vi "PCO_CheckDeviceAvailability.vi"(8 "error in (no error)":errorcluster {"code" format="%x"}, 10 "wNum":u16, 11 "ph":u64) -> (0 "error out":errorcluster {"code" format="%x"}, 2 "ErrorMessage":i32 format="%x", 3 "ph out":u64)   [LabVIEW 2019, in "SDK.lvlib" / "CameraAccess.lvlib"]
doc: "<b>Description:</b>\nThis function is used to check, if the connection to a previously opened camera is still valid. Functionality is only supported for interfaces with HotPlug capability like USB, GigE or FireWire.\nIf a device is connected or disconnected from a HotPlug capable bus system, the device manager does invoke a bus reset call on the bus and afterwards is starting a new enumeration. If enumeration is finished, a DEVICE_CHANGE message is broadcasted to all applications.\n\n<b>Supported camera type:</b>\nInterface dependent\n\n<b>Descriptor dependency:</b>\nNone"
uses:
  CameraAccess.lvlib
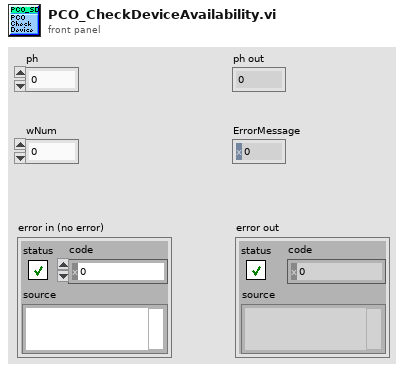
[diagram p1: front panel]
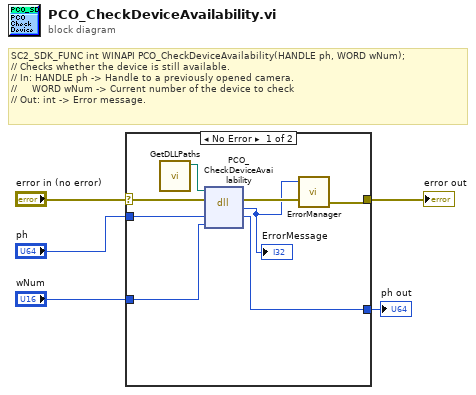
[diagram p0: block diagram]
diagram:
  # "SC2_SDK_FUNC int WINAPI PCO_CheckDeviceAvailability(HANDLE ph, WORD wNum);\n// Checks whether the device is still available.\n// In: HANDLE ph -> Handle to a previously opened camera.\n//     WORD wNum -> Current number of the device to check\n// Out: int -> Error message."
  n1 = case shown="No Error" "error in (no error)" {
    selector: "error in (no error)" -> [w12 w15]
    tunnel: [w13 w15] -> w5
    tunnel: [w9 w14] -> w3
    tunnel: "ph" -> [w8 w14]
    tunnel: "wNum" -> [w7 _]
    frame No Error {
      n2 = call "GetDLLPaths.vi"() -> ("SC2_Cam_Path"=w6:path)  [unwired: 8 in, 3 out]
      n3 = dll-call lib="?" fn="PCO_CheckDeviceAvailability"(path in=w6, error in=w12, "ph"=w8, "wNum"=w7) -> (error out=w11:errorcluster, "return type"=w10:i32, "ph"=w9:u64)  [unwired: 2 in, 1 out]
      "ErrorMessage" <- w10
      n4 = call "ErrorManager.vi"("error in (no error)"=w11, "error code"=w10) -> ("error out"=w13:errorcluster)  [unwired: 2 in, 1 out]
    }
    frame Error {
    }
  }
  "error out" <- w5
  "ph out" <- w3
